vi "Text Ring to Caption and String[ ].vi"(8 "Numeric (0)":u8, 11 "String":string) -> (1 "String[ ]":string[](array[string]), 3 "Caption":string)   [LabVIEW 2013, in "main.lvlib"]
doc: "Jean-Marc Simard \nExaprom inc. 2009"
uses:
  main.lvlib
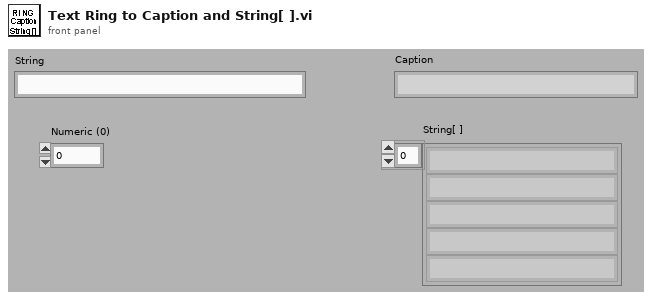
[diagram p1: front panel]
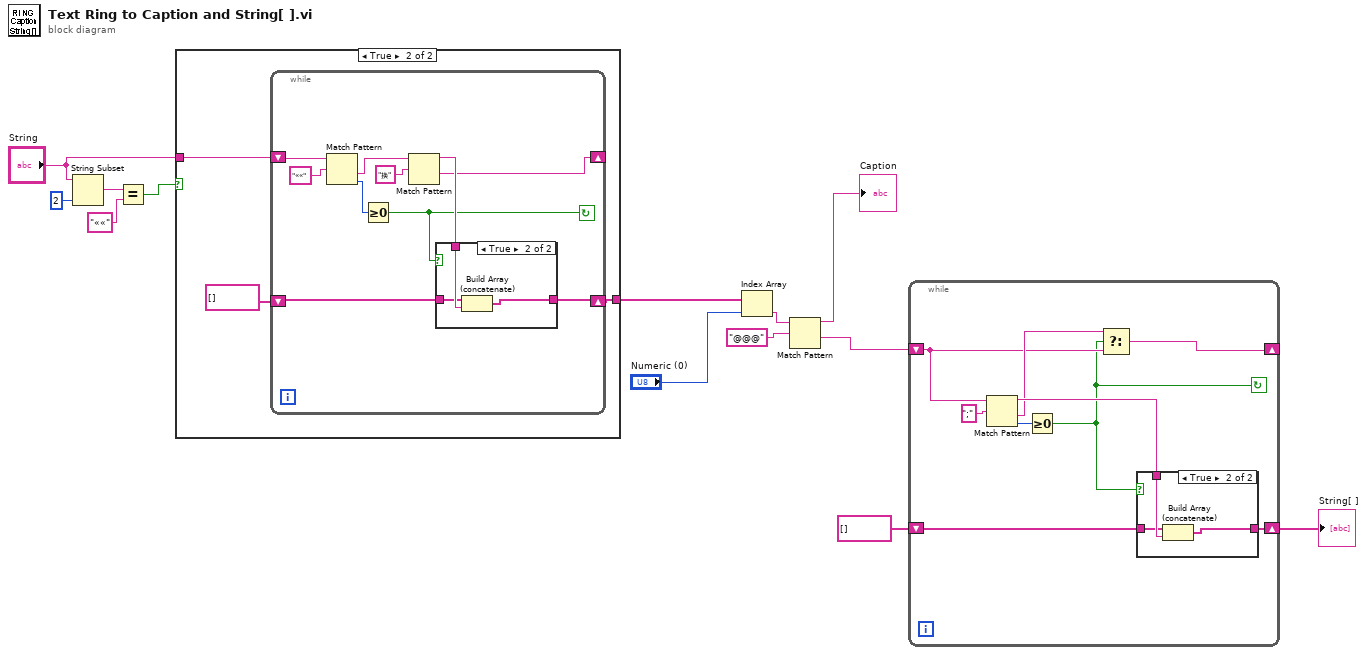
[diagram p0: block diagram]
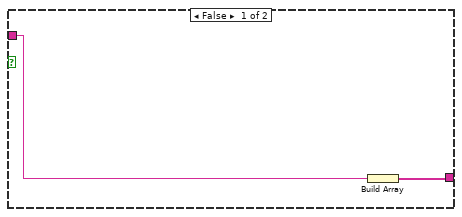
[diagram p2: hidden frame]
diagram:
  n1 = String Subset(string="String", length (rest)=2 ("length (rest)")) -> (substring=w7:string)  [unwired: 1 out]
  n2 = Equal?(x=w7, y="««") -> (x = y?=w5:bool)
  n3 = case shown="True" w5 {
    tunnel: "String" -> [w15 w18]
    tunnel: [w14 w16] -> w3
    frame False {
      n4 = Build Array(w15) -> (w14:string[])
    }
    frame True {
      n5 = while {
        shift-right: [w21] -> _
        shift-left: w18 -> [w25]
        shift-right: [w24] -> w16
        shift-left: string[] [] ("String[ ]") -> [w23]
        stop <- w19 continue-if-true
        n6 = Match Pattern(string=w25, regular expression="««" ("y")) -> (after substring=w27:string, offset past match=w20:i32)  [unwired: 3 out]
        n7 = Greater Or Equal To 0?(x=w20) -> (x >= 0?=w19:bool)
        n8 = Match Pattern(string=w27, regular expression="换" ("y")) -> (before substring=w22:string, after substring=w21:string)  [unwired: 3 out]
        n9 = case shown="True" w19 {
          tunnel: w22 -> [_ w32]
          tunnel: w23 -> [w29 w31]
          tunnel: [w29 w30] -> w24
          frame False {
          }
          frame True {
            n10 = Build Array (concatenate)(w31, w32) -> (w30:string[])
          }
        }
      }
    }
  }
  n11 = Index Array(array=w3, index="Numeric (0)") -> (element=w2:string)
  n12 = Match Pattern(string=w2, regular expression="@@@") -> (before substring=→"Caption":string, after substring=w11:string)  [unwired: 3 out]
  n13 = while {
    shift-right: [w39] -> _
    shift-left: w11 -> [w34]
    shift-right: [w36] -> w9
    shift-left: string[] [] ("String[ ]") -> [w37]
    stop <- w33 continue-if-true
    n14 = Match Pattern(string=w34, regular expression=";") -> (before substring=w38:string, after substring=w35:string, offset past match=w40:i32)  [unwired: 2 out]
    n15 = Greater Or Equal To 0?(x=w40) -> (x >= 0?=w33:bool)
    n16 = Select(t=w35, s=w33, f=w34) -> (s? t:f=w39:string)
    n17 = case shown="True" w33 {
      tunnel: w38 -> [_ w45]
      tunnel: w37 -> [w42 w44]
      tunnel: [w42 w43] -> w36
      frame False {
      }
      frame True {
        n18 = Build Array (concatenate)(w44, w45) -> (w43:string[])
      }
    }
  }
  "String[ ]" <- w9
